vi "Benchmark SV Receive LV2012 - NI Verified - 10 Byte.vi"() -> ()   [LabVIEW 2015]
panel:
  in  "10 byte 2":u64[][](array[numeric])=[[0, 0, 0, 0, 0, 0, 0, 0, 0, 0], [0, 0, 0, 0, 0, 0, 0, 0, 0, 0]]
  out "appended array":u64[][](array[numeric])
  out "10 byte":u64[](array[numeric])
  in  "stop":bool
  # "Overview:  Coding that exemplifies how to benchmark the communication of Shared Variables.\nRequirements: LabVIEW 2012 or compatible\nInstructions:\n1. Run this VI\n2. Watch the amount of time it takes to communicate on the \"Benchmark SV Send  LV2012 - NI Verified.vi\" \n3. Stop both VIs"
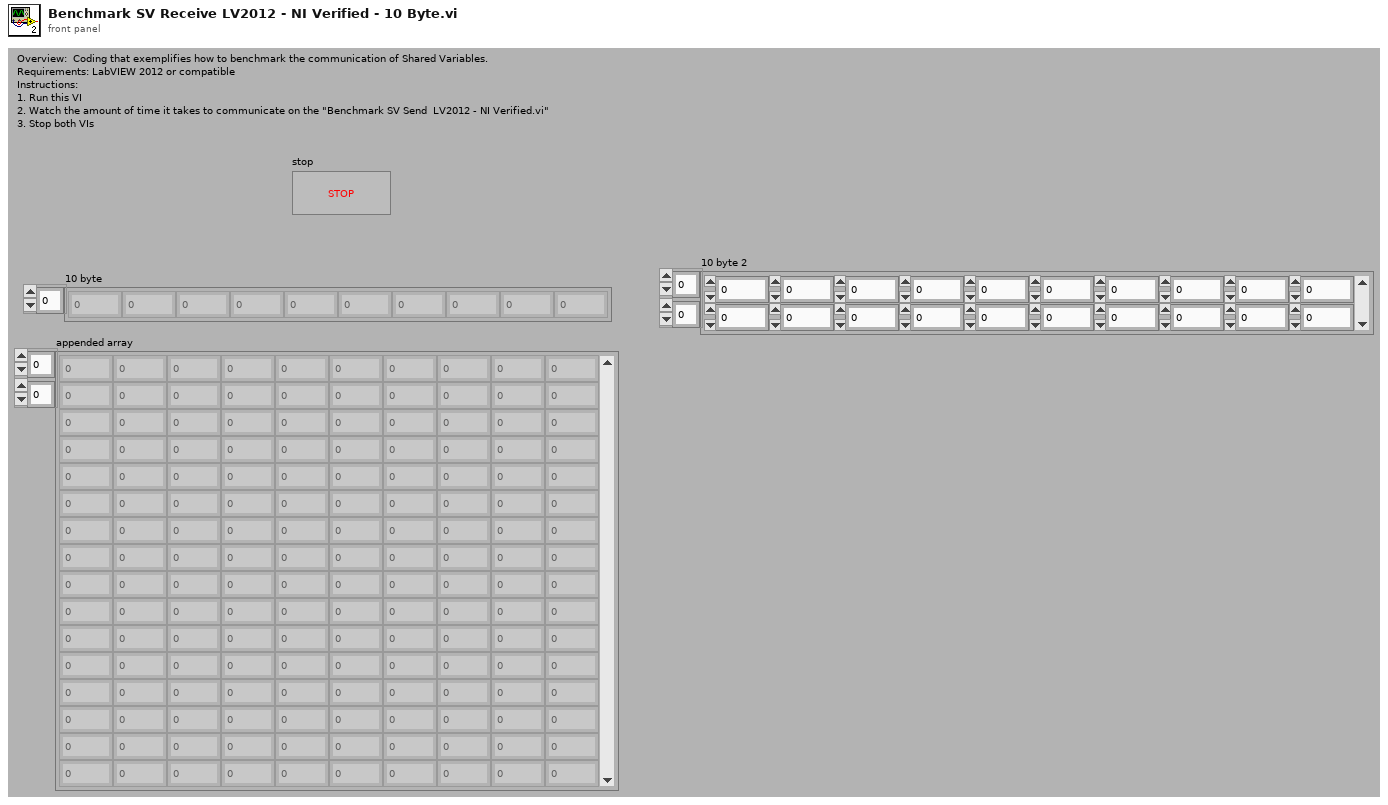
[diagram p1: front panel]
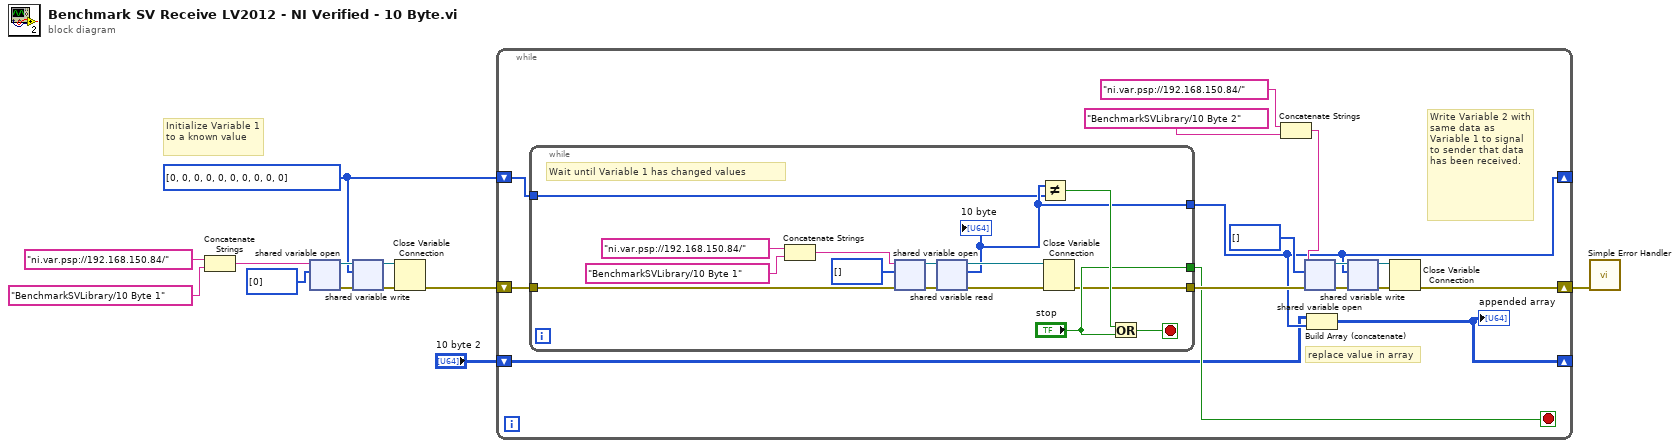
[diagram p0: block diagram]
diagram:
  w2 = u64[] [0, 0, 0, 0, 0, 0, 0, 0, 0, 0] ("appended array")
  # "Initialize Variable 1 to a known value"
  n1 = Concatenate Strings("ni.var.psp://192.168.150.84/" ("string"), "BenchmarkSVLibrary/10 Byte 1") -> (w11:string)
  n2 = shared-variable-open(w11, u64[] [0] ("appended array")) -> (w9:refnum<k21>, w7:errorcluster)  [unwired: 2 in]
  n3 = shared-variable-write(w9, w7, w2) -> (w8:refnum<k21>, w6:errorcluster)
  n4 = Close Variable Connection(8:w6, 11:w8) -> (0:w5:errorcluster)
  n5 = while {
    shift-right: [w15] -> _
    shift-left: w2 -> [w28]
    shift-right: [w17] -> w12
    shift-left: w5 -> [w27]
    shift-right: [w14] -> _
    shift-left: "10 byte 2" -> [w13]
    stop <- w16 stop-if-true
    # "replace value in array"
    # "Write Variable 2 with same data as Variable 1 to signal to sender that data has been received."
    n6 = while {
      tunnel: w28 -> [w29]
      tunnel: [w30] -> w15
      tunnel: ["stop"] -> w16
      tunnel: [w35] -> w18
      tunnel: w27 -> [w34]
      stop <- w41 stop-if-true
      # "Wait until Variable 1 has changed values"
      n7 = Concatenate Strings("ni.var.psp://192.168.150.84/" ("string"), "BenchmarkSVLibrary/10 Byte 1") -> (w31:string)
      n8 = shared-variable-open(w31, w34, u64[] [] ("appended array")) -> (w39:refnum<k21>, w38:errorcluster)  [unwired: 1 in]
      n9 = shared-variable-read(w39, w38) -> (w37:refnum<k21>, w36:errorcluster, w30:u64[])  [unwired: 1 out]
      "10 byte" <- w30
      n10 = Not Equal?(x=w30, y=w29) -> (x != y?=w43:bool)
      n11 = Close Variable Connection(8:w36, 11:w37) -> (0:w35:errorcluster)
      n12 = Or(x=w43, y="stop") -> (x .or. y?=w41:bool)
    }
    n13 = Concatenate Strings("ni.var.psp://192.168.150.84/" ("string"), "BenchmarkSVLibrary/10 Byte 2") -> (w25:string)
    n14 = shared-variable-open(w25, w18, u64[] [] ("appended array")) -> (w24:refnum<k21>, w23:errorcluster)  [unwired: 1 in]
    n15 = Build Array (concatenate)(w13, w15) -> (w14:u64[][])
    "appended array" <- w14
    n16 = shared-variable-write(w24, w23, w15) -> (w22:refnum<k21>, w21:errorcluster)
    n17 = Close Variable Connection(8:w21, 11:w22) -> (0:w17:errorcluster)
  }
  n18 = call <vilib>:"Simple Error Handler.vi"("error in (no error)"=w12) -> ()  [unwired: 4 in, 5 out]
